vi "write file header.vi"(3 "refnum":refnum<file>) -> (1 "dup refnum":refnum<file>)   [LabVIEW 2012]
uses:
  calibration/global scale array.vi
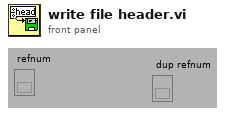
[diagram p1: front panel]
types:
  T1 = typedef "calib array.ctl" = T2[]
  T2 = typedef "conversion.ctl" = cluster{"conversion matrix":sgl[][], "units":string, "name":string, "scale type":T3, "offset (volts)":dbl, "second channel":i8, "correspondence table":T4, "offset (physical units)":dbl, "pH scale":T5, "D.O.":T6}
  T3 = typedef "scale type.ctl" = enum16{"Volts", "Polynomial", "Correspondence Table", "pH", "Dissolved Oxygen", "Quadratic"}
  T4 = typedef "correspondence table.ctl" = cluster{"physical units":dbl, "volts":dbl}[]
  T5 = typedef "pH scale.ctl" = cluster{"Buffers":cluster{"Buffer":dbl, "Calibrated":bool, "V/T":dbl}[], "Temperature":dbl}
  T6 = typedef "DO scale.ctl" = cluster{"Temperature":dbl, "K":dbl, "barometric pressure":dbl}
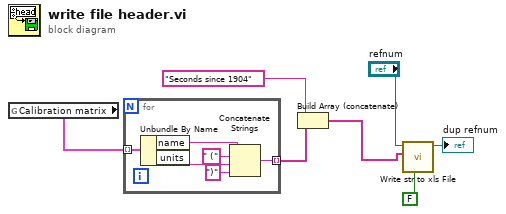
[diagram p0: block diagram]
diagram:
  n1 = global read "global scale array.vi" "Calibration matrix"() -> (w4:T1)
  n2 = for {
    tunnel: w4 -> [w13] mode=indexing
    tunnel: [w8] -> w3 mode=indexing
    n3 = Unbundle By Name(w13) -> ("name"=w12:string, "units"=w10:string)
    n4 = Concatenate Strings(w12, " (" ("string"), w10, ")" ("string")) -> (w8:string)
  }
  n5 = Build Array (concatenate)("Seconds since 1904", w3) -> (w1:string[])
  n6 = call "Write str to xls File.vi"("transpose? (no:F)"=FALSE, "1D data"=w1, "refnum"="refnum") -> ("dup refnum"=→"dup refnum":refnum<file>)  [unwired: 7 in, 1 out]
